vi "20211022_HW03.vi"() -> ()   [LabVIEW 2019]
panel:
  out "Result":string
  in  "Text":string
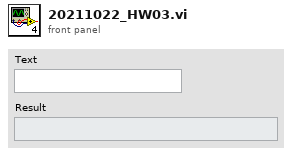
[diagram p1: front panel]
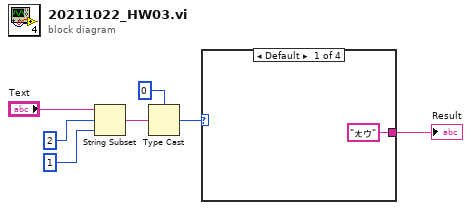
[diagram p0: block diagram]
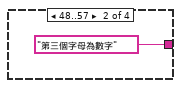
[diagram p2: hidden frame]
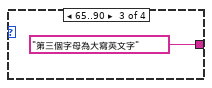
[diagram p3: hidden frame]
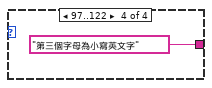
[diagram p4: hidden frame]
diagram:
  n1 = String Subset(string="Text", offset (0)=2, length (rest)=1 ("length (rest)")) -> (substring=w4:string)
  n2 = Type Cast(type=u8 0, x=w4) -> (*(type *) &x=w2:u8)
  n3 = case shown="Default" w2 {
    tunnel: ["ㄤウ" ("Result") "第三個字母為數字" ("Result") "第三個字母為大寫英文字" ("Result") "第三個字母為小寫英文字" ("Result")] -> w1
    frame Default {
    }
    frame 48..57 {
    }
    frame 65..90 {
    }
    frame 97..122 {
    }
  }
  "Result" <- w1
